vi "Keithley2100.measure AC voltage.vi"(0 "i ref in":refnum<vi>, 1 "Custom Range (100mV)":dbl=0.1 min=0.1 max=1000.0 format="%#.6e", 2 "Digital Filter (0: Off)":u16(ring) items=["Off", "Moving Filter", "Repeating Filter"], 3 "Digital Filter Readings (10)":i32=10, 4 "NPLC":u16(ring)=2 items=[".02", ".1", "1", "10"], 5 "error in (no error)":errorcluster, 9 "Auto Range":bool) -> (14 "i refout":refnum<vi>, 16 "Measurement":dbl format="%#_6e", 19 "error out":errorcluster)   [LabVIEW 2014, in "Keithley2100.lvlib"]
doc: "This VI is used to get the USB port of the USBSwitchBox from the database.\n\nLicense Agreement for this software:\n\nCopyright (C)\nGesellschaft für Schwerionenforschung, GSI\nPlanckstr. 1\n64291 Darmstadt\nGermany\n\nContact: D.Beck@gsi.de \n\nThis program is free software; you can redistribute it and/or modify it under the terms of the \nGNU General Public License as published by the Free Software Foundation; either version 2 of \nthe license, or (at your option) any later version.\n\nThis program is distributed in the hope that it will be useful, but WITHOUT ANY WARRANTY; \nwithout even the implied warranty of MERCHANTABILITY or FITNESS FOR A PARTICULAR PURPOSE. See the GNU General License for more details (http://www.gnu.org).\n\nGesellschaft für Schwerionenforschung, GSI\nPlanckstr. 1, 64291 Darmstadt, Germany\nFor all questions and ideas contact: M.Richter@gsi.de, H.Brand@gsi.de or D.Beck@gsi.de.\nLast update: 16-JUN-2004"
uses:
  Keithley2100.lvlib
  instr.lib/Keithley-2100-Series/Keithley 2100 Series.lvlib
  CSlibraries-extern/DimLVEvent/LVDimInterface/LVDimInterface.lvlib
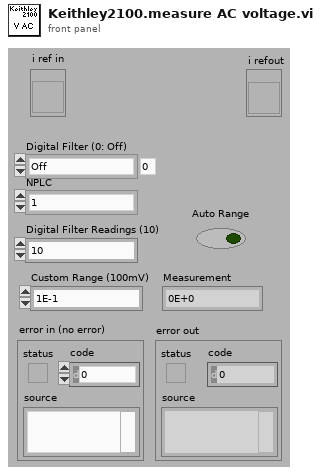
[diagram p1: front panel]
types:
  T1 = typedef "Keithley2100.lvlib/Keithley2100.i attribute.ctl" = cluster{"Custom Range":dbl, "Threshold Range":dbl, "VISA resource name":refnum<visa-resource-name>, "Auto Range":bool, "Digital Filter Readings":i32, "Digital Filter":u16, "NPLC":u16, "Display on":u16, "Resolution":u16, "Beaper enabled":bool, "MeasurementID":i32}
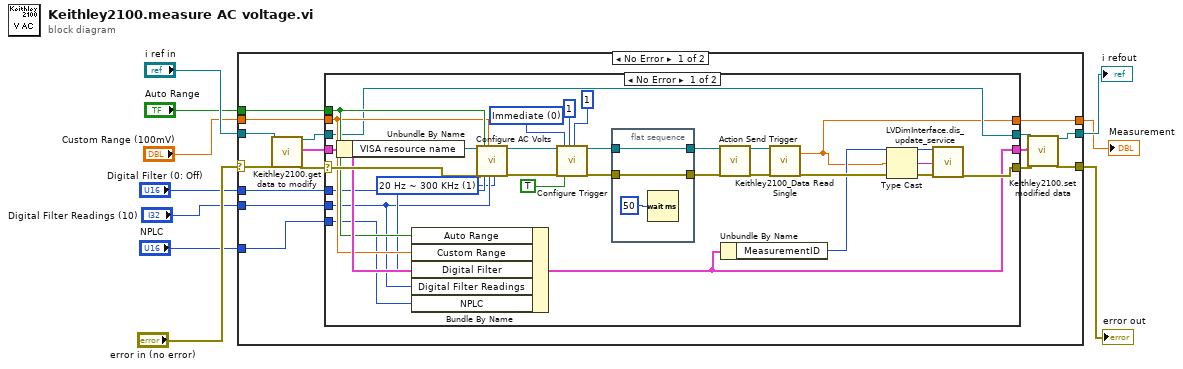
[diagram p0: block diagram]
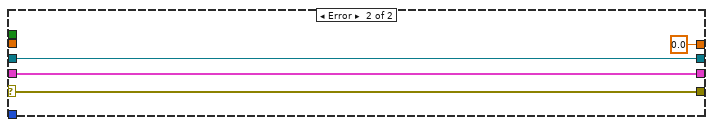
[diagram p2: hidden frame]
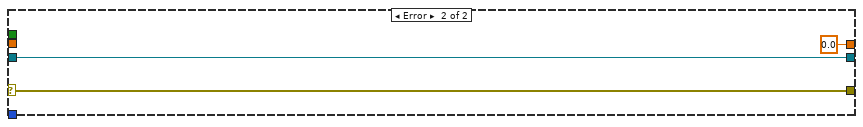
[diagram p3: hidden frame]
diagram:
  n1 = case shown="No Error" "error in (no error)" {
    selector: "error in (no error)" -> [w25 w64]
    tunnel: [w20 w64] -> w8
    tunnel: "i ref in" -> [w26 w63]
    tunnel: [w21 w63] -> w7
    tunnel: "Auto Range" -> [w16 _]
    tunnel: "Custom Range (100mV)" -> [w15 _]
    tunnel: "Digital Filter (0: Off)" -> [w14 _]
    tunnel: "Digital Filter Readings (10)" -> [w13 _]
    tunnel: "NPLC" -> [w12 _]
    tunnel: [w11 0.0 ("Measurement")] -> w1
    frame No Error {
      n2 = call "Keithley2100.get data to modify.vi"("i ref in"=w26, "error in (no error)"=w25) -> ("i ref out"=w23:refnum<vi>, "i attribute"=w22:T1, "error out"=w24:errorcluster)  [unwired: 14 in, 1 out]
      n3 = case shown="No Error" w24 {
        selector: w24 -> [w53 w60]
        tunnel: w23 -> [w34 w61]
        tunnel: w22 -> [w52 w59]
        tunnel: [w34 w61] -> w19
        tunnel: [w32 w60] -> w18
        tunnel: [w31 w59] -> w17
        tunnel: w16 -> [w51 _]
        tunnel: w15 -> [w50 _]
        tunnel: w14 -> [w49 _]
        tunnel: w13 -> [w48 _]
        tunnel: w12 -> [w47 _]
        tunnel: [w29 0.0 ("Measurement")] -> w11
        frame No Error {
          w27 = u16 1 items=["3 Hz ~ 300 KHz", "20 Hz ~ 300 KHz", "200 Hz ~ 300 KHz"] ("Bandwidth (20 Hz)")
          w42 = u16 0 items=["Immediate", "Bus", "External"] ("Source (0: Immediate)")
          n4 = Unbundle By Name(w52) -> ("VISA resource name"=w54:refnum<visa-resource-name>)
          n5 = Bundle By Name(cluster=w52, "Auto Range"=w51, "Custom Range"=w50, "Digital Filter"=w49, "Digital Filter Readings"=w48, "NPLC"=w47) -> (w31:T1)
          n6 = call "Configure AC Volts.vi"("VISA resource name"=w54, "error in (no error)"=w53, "Auto Range? (T: Auto)"=w51, "Digital Filter (0: Off)"=w49, "Custom Range (0 V)"=w50, "Digital Filter Readings (10)"=w48, "Bandwidth (20 Hz)"=w27) -> ("VISA resource name out"=w46:refnum<visa-resource-name>, "error out"=w45:errorcluster)  [unwired: 11 in]
          n7 = call "Configure Trigger.vi"("VISA resource name"=w46, "error in (no error)"=w45, "Source (0: Immediate)"=w42, "Auto Delay? (T: Auto)"=TRUE, "Sample Count (1)"=1, "Trigger Count (1)"=1) -> ("VISA resource name out"=w40:refnum<visa-resource-name>, "error out"=w39:errorcluster)  [unwired: 12 in]
          n8 = flat-sequence {
            tunnel: [w56] -> w38
            tunnel: w40 -> [w56]
            tunnel: [w55] -> w37
            tunnel: w39 -> [w55]
            frame #0 {
              n9 = Wait (ms)(milliseconds to wait=u32 50) -> ()  [unwired: 1 out]
            }
          }
          n10 = call "Action Send Trigger.vi"("VISA resource name"=w38, "error in (no error)"=w37) -> ("VISA resource name out"=w36:refnum<visa-resource-name>, "error out"=w35:errorcluster)  [unwired: 16 in]
          n11 = Unbundle By Name(w31) -> ("MeasurementID"=w30:i32)
          n12 = call "Keithley2100_Data Read Single.vi"("VISA resource name"=w36, "error in (no error)"=w35) -> ("Measurement"=w29:dbl, "error out"=w33:errorcluster)  [unwired: 15 in, 1 out]
          n13 = Type Cast(x=w29) -> (*(type *) &x=w28:string)  [unwired: 1 in]
          n14 = call "LVDimInterface.dis_update_service.vi"("my_serviceID"=w30, "data"=w28, "error in (no error)"=w33) -> ("error out"=w32:errorcluster)  [unwired: 14 in, 2 out]
        }
        frame Error {
        }
      }
      n15 = call "Keithley2100.set modified data.vi"("i ref in"=w19, "i attribute"=w17, "error in (no error)"=w18) -> ("i ref out"=w21:refnum<vi>, "error out"=w20:errorcluster)  [unwired: 15 in]
    }
    frame Error {
    }
  }
  "error out" <- w8
  "i refout" <- w7
  "Measurement" <- w1
